vi "Update Output Latch.vi"   [LabVIEW 2014, in "MCP23S17.lvlib"]
doc: "Update the output latch of the pins."
uses:
  MCP23S17.lvlib
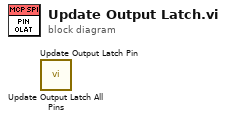
[diagram p0: block diagram]
diagram:
  n1 = call "Update Output Latch All Pins.vi"() -> ()  [unwired: 9 in, 3 out]
  n2 = call "Update Output Latch Pin.vi"() -> ()  [unwired: 9 in, 3 out]
